vi "Parse Project for DQMH Modules.vi"(0 "Project (unwired: Active Project)":refnum<vi>, 5 "Allowable Module Type":T2(ring), 11 "error in (no error)":errorcluster) -> (3 "project owning folder":path, 4 "DQMH Modules":T1(array[cluster]), 8 "My Computer":refnum<vi>, 10 "Any Dirty Modules?":bool, 13 "All Libraries in Project":string[](array[string]), 14 "Any Locked Modules?":bool, 15 "error out":errorcluster)   [LabVIEW 2016, in "DQMH_API.lvclass"]
uses:
  <resource>/Framework/Providers/Open_GDS/UML/DQMH_API_class/DQMH_API.lvclass
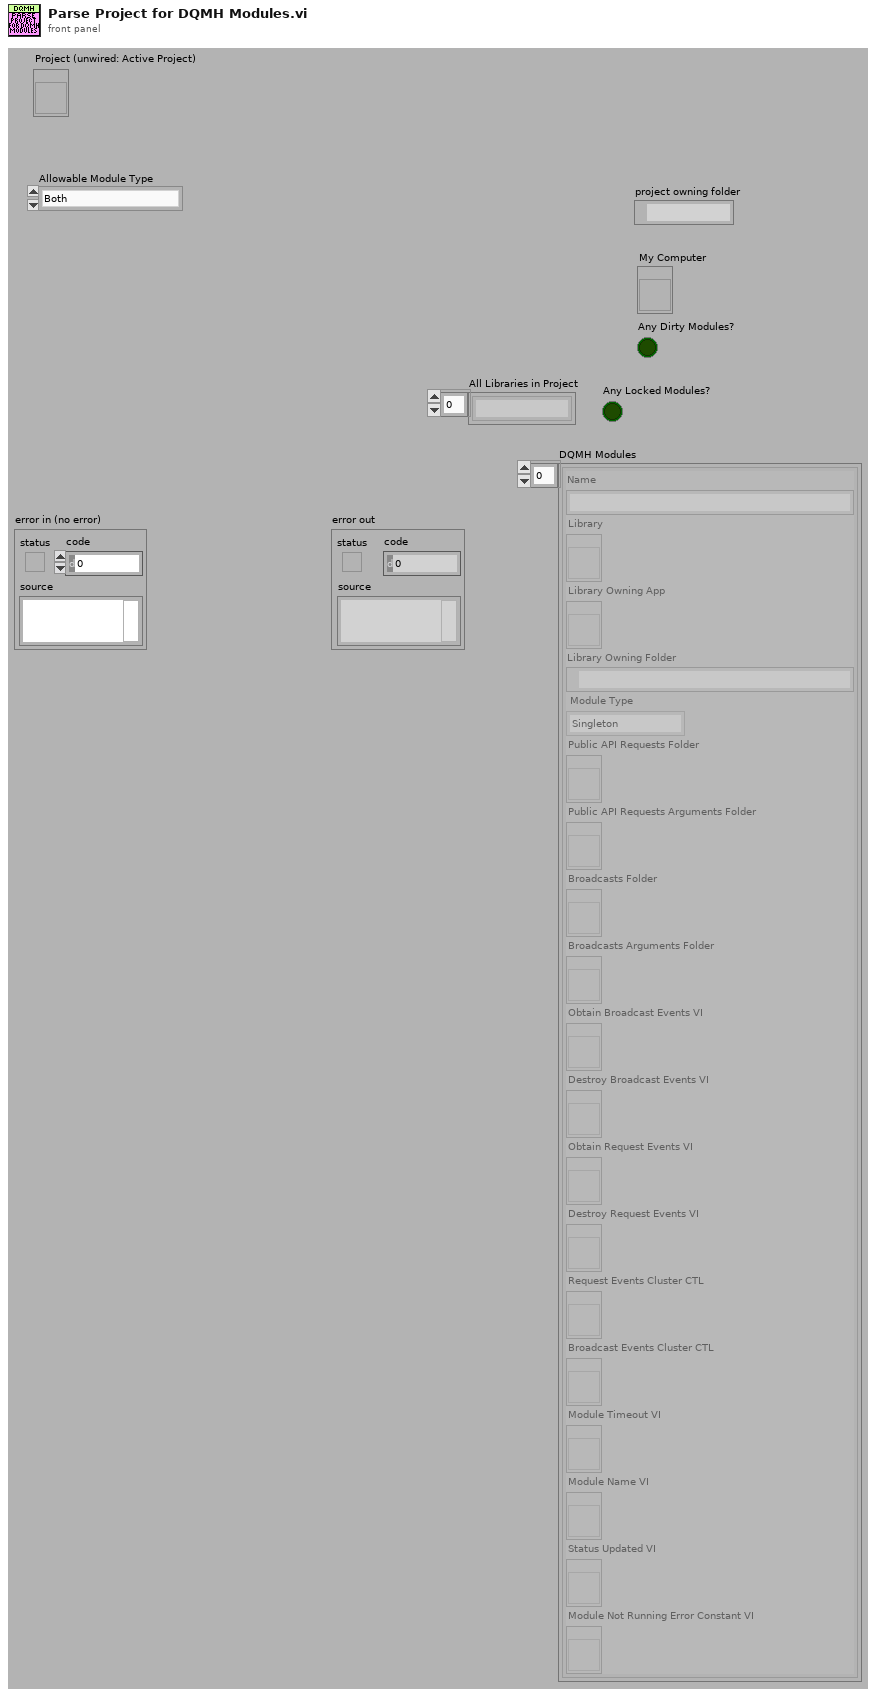
[diagram p1: front panel]
types:
  T1 = cluster{"Name":string, "Library":refnum<vi>, "Library Owning App":refnum<vi>, "Library Owning Folder":path, "Module Type":enum16{"Singleton", "Cloneable"}, "Public API Requests Folder":refnum<vi>, "Public API Requests Arguments Folder":refnum<vi>, "Broadcasts Folder":refnum<vi>, "Broadcasts Arguments Folder":refnum<vi>, "Obtain Broadcast Events VI":refnum<vi>, "Destroy Broadcast Events VI":refnum<vi>, "Obtain Request Events VI":refnum<vi>, "Destroy Request Events VI":refnum<vi>, "Request Events Cluster CTL":refnum<vi>, "Broadcast Events Cluster CTL":refnum<vi>, "Module Timeout VI":refnum<vi>, "Module Name VI":refnum<vi>, "Status Updated VI":refnum<vi>, "Module Not Running Error Constant VI":refnum<vi>}[]
  T2 = enum16{"Both", "Singleton Only", "Cloneable Only"}
  T3 = typedef "DQMH_API.lvclass/ObjectAttributes.ctl" = cluster{"Get Module Type Info":refnum<vi>, "Script New Module":refnum<vi>, "Script New Event":refnum<vi>, "Query Library for Module Info":refnum<vi>, "Parse Project for DQMH Modules":refnum<vi>, "Get All Events in Module":refnum<vi>}
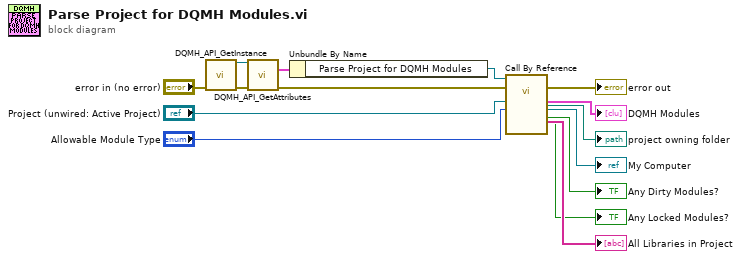
[diagram p0: block diagram]
diagram:
  n1 = call <resource>:"DQMH_API_GetInstance.vi"("error in (no error)"="error in (no error)") -> ("reference out"=w12:refnum<class "DQMH_API.lvclass">, "error out"=w11:errorcluster)  [unwired: 10 in, 3 out]
  n2 = call <resource>:"DQMH_API_GetAttributes.vi"("reference in"=w12, "error in (no error)"=w11) -> ("Data"=w13:T3, "error out"=w9:errorcluster)  [unwired: 10 in, 2 out]
  n3 = Unbundle By Name(w13) -> ("Parse Project for DQMH Modules"=w10:refnum<vi>)
  n4 = call-by-ref "?"(reference=w10, error in=w9, "Allowable Module Type"="Allowable Module Type", "Project (unwired: Active Project)"="Project (unwired: Active Project)") -> (error out=→"error out":errorcluster, "Any Dirty Modules?"=→"Any Dirty Modules?":bool, "My Computer"=→"My Computer":refnum<vi>, "DQMH Modules"=→"DQMH Modules":T1, "Any Locked Modules?"=→"Any Locked Modules?":bool, "project owning folder"=→"project owning folder":path, "All Libraries in Project"=→"All Libraries in Project":string[])  [unwired: 3 in, 2 out]
